vi "Public Get Error Handler.vi"(8 "error in (no error)":errorcluster, 11 "Mock Process in":refnum<class "Mock Process.lvclass">) -> (0 "error out":errorcluster, 2 "Error Handler":refnum<class "Error Handler Interface.lvclass">, 3 "Mock Process out":refnum<class "Mock Process.lvclass">)   [LabVIEW 2020, in "Mock Process.lvclass"]
uses:
  Mock Process.lvclass
  Framework/Error Handler Interface/Error Handler Interface.lvclass
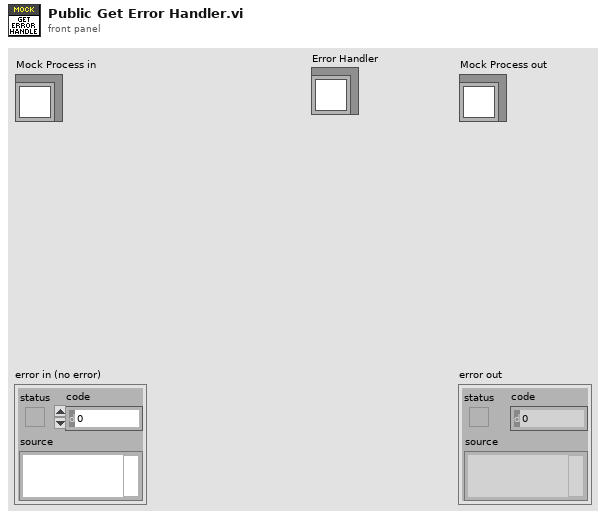
[diagram p1: front panel]
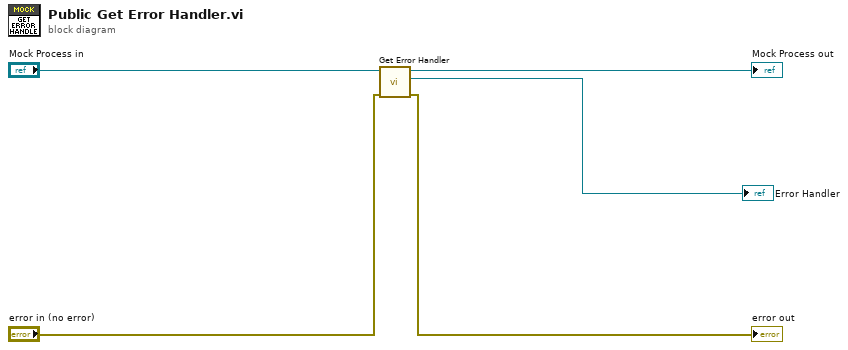
[diagram p0: block diagram]
diagram:
  n1 = call-dynamic "Get Error Handler.vi"("error in (no error)"="error in (no error)", "Process In"="Mock Process in") -> ("error out"=→"error out":errorcluster, "Error Handler"=→"Error Handler":refnum<class "Error Handler Interface.lvclass">, "Process Out"=→"Mock Process out":refnum<class "Mock Process.lvclass">)  [unwired: 7 in]
